vi "Aggregate Suite Result.vi"(8 "error in (no error)":errorcluster, 10 "Test Suite Result":T1, 11 "Report In":refnum<class "Test Report.lvclass">) -> (0 "error out":errorcluster, 3 "Report Out":refnum<class "Test Report.lvclass">)   [LabVIEW 2020, in "Test Report.lvclass"]
uses:
  Test Report.lvclass
  Result Types/Suite Results/Test Suite Result.ctl
  Core/Result/Status.ctl
  Result Types/Case Result/Test Case Result.ctl
  Result Types/Method Result/Method Result.ctl
  Result Types/Assertion Result/Assertion Result.ctl
  Result Types/Assertion Result/Public/TypeDefs/Assertion Type.ctl
  Test Report.lvclass/Test Report.ctl
  Result Types/Suite Results/Private/Count by Status.vi
  Result Types/Case Result/Public/Read Status.vi
  Result Types/Case Result/Private/Merge Status.vi
  Result Types/Method Result/Public/Read Status.vi
  Result Types/Suite Results/Test Suite Result.lvlib
  Result Types/Assertion Result/Assertion Result.lvlib
  Result Types/Method Result/Method Result.lvlib
  Result Types/Case Result/Test Case Result.lvlib
  Core/Result/Result.lvlib
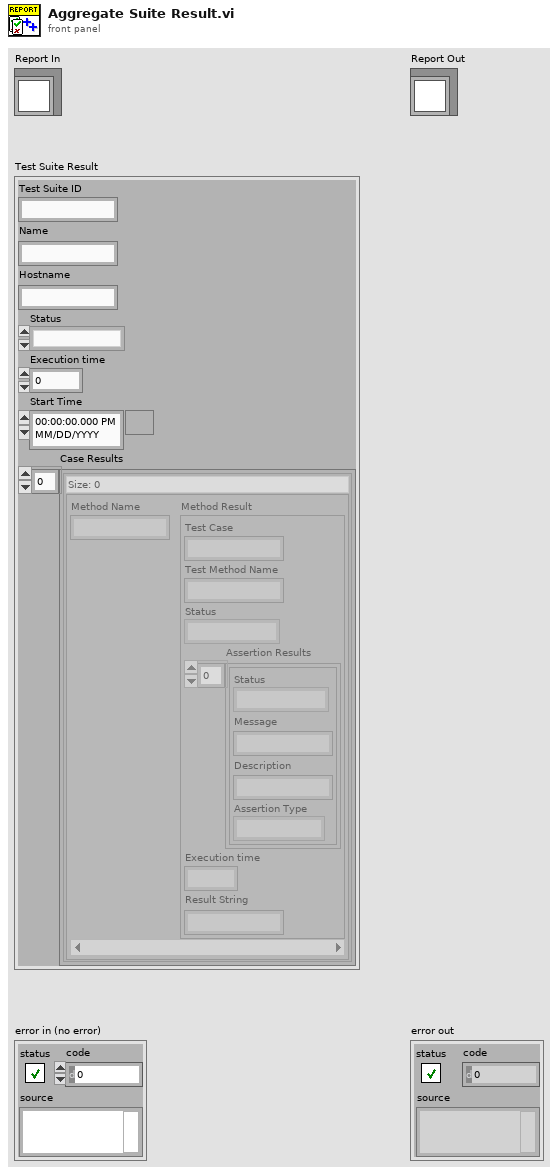
[diagram p1: front panel]
types:
  T1 = typedef "Test Suite Result.lvlib/Test Suite Result.ctl" = cluster{"Test Suite ID":string, "Name":string, "Hostname":string, "Status":T2, "Execution time":dbl, "Start Time":timestamp, "Case Results":T3[]}
  T2 = typedef "Result.lvlib/Status.ctl" = enum16{"", "Passed", "Failed", "Error", "Skipped", "Setup Error", "Broken", "Teardown Error"}
  T3 = typedef "Test Case Result.lvlib/Test Case Result.ctl" = map{string, T4}
  T4 = typedef "Method Result.lvlib/Method Result.ctl" = cluster{"Test Case":string, "Test Method Name":string, "Status":T2, "Assertion Results":T5[], "Execution time":dbl, "Result String":string}
  T5 = typedef "Assertion Result.lvlib/Assertion Result.ctl" = cluster{"Status":T2, "Message":string, "Description":string, "Assertion Type":T6}
  T6 = typedef "Result.lvlib/Assertion Type.ctl" = enum16{"None", "Pass", "Fail", "Skip", "Pass if Equal", "Fail if Equal", "Pass if Error", "Fail if Error", "Pass if", "Fail if"}
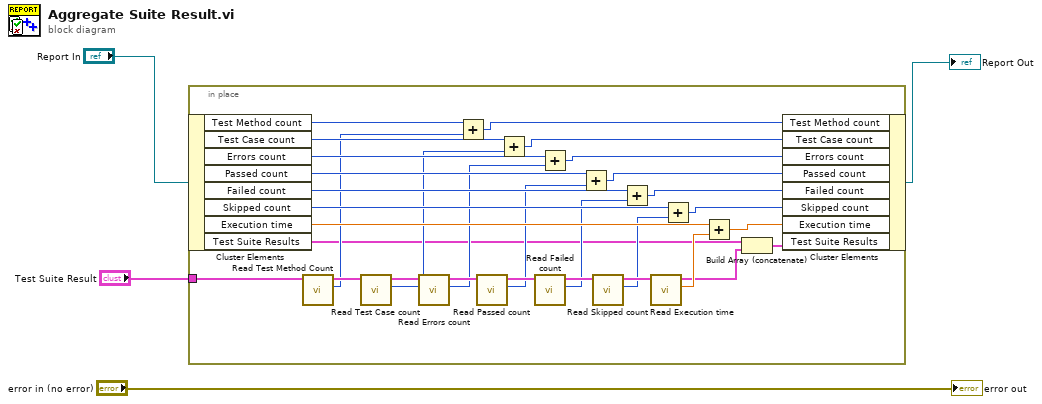
[diagram p0: block diagram]
diagram:
  n1 = in-place {
    in-place-border: "Test Suite Result" -> [w22]
    n2 = in-place-cluster #1("Report In") -> ("Test Method count"=w35:i32, "Test Case count"=w34:i32, "Errors count"=w33:i32, "Passed count"=w32:i32, "Failed count"=w29:i32, "Skipped count"=w31:i32, "Execution time"=w30:dbl, "Test Suite Results"=w7:T1[])
    n3 = call "Read Test Method Count.vi"("Test Suite Result In"=w22) -> ("Test Method count"=w15:i32, "Test Suite Result Out"=w28:T1)  [unwired: 8 in, 1 out]
    n4 = call "Read Test Case count.vi"("Test Suite Result In"=w28) -> ("Test Case count"=w16:i32, "Test Suite Result Out"=w27:T1)  [unwired: 9 in]
    n5 = call "Read Errors count.vi"("Test Suite Result In"=w27) -> ("Errors count"=w17:i32, "Test Suite Result Out"=w26:T1)  [unwired: 8 in, 1 out]
    n6 = Add(x=w35, y=w15) -> (x+y=w8:i32)
    n7 = call "Read Passed count.vi"("Test Suite Result In"=w26) -> ("Pass count"=w18:i32, "Test Suite Result Out"=w25:T1)  [unwired: 9 in]
    n8 = Add(x=w34, y=w16) -> (x+y=w9:i32)
    n9 = call "Read Failed count.vi"("Test Suite Result In"=w25) -> ("Failures count"=w19:i32, "Test Suite Result Out"=w24:T1)  [unwired: 8 in, 1 out]
    n10 = Add(x=w33, y=w17) -> (x+y=w10:i32)
    n11 = Add(x=w32, y=w18) -> (x+y=w11:i32)
    n12 = call "Read Skipped count.vi"("Test Suite Result In"=w24) -> ("Skipped count"=w20:i32, "Test Suite Result Out"=w23:T1)  [unwired: 8 in, 1 out]
    n13 = Add(x=w29, y=w19) -> (x+y=w12:i32)
    n14 = call "Read Execution time.vi"("Test Suite Result In"=w23) -> ("Execution time"=w21:dbl, "Test Suite Result Out"=w5:T1)  [unwired: 8 in, 1 out]
    n15 = Add(x=w31, y=w20) -> (x+y=w13:i32)
    n16 = Add(x=w30, y=w21) -> (x+y=w14:dbl)
    n17 = Build Array (concatenate)(w7, w5) -> (w6:T1[])
    n18 = in-place-cluster #1("Test Method count"=w8, "Test Case count"=w9, "Errors count"=w10, "Passed count"=w11, "Failed count"=w12, "Skipped count"=w13, "Execution time"=w14, "Test Suite Results"=w6) -> (→"Report Out":refnum<class "Test Report.lvclass">)
  }
  "error out" <- "error in (no error)"
